vi "Mensagem.vi"(2 "error in (no error)":errorcluster, 3 "tamanho":i32) -> (0 "error IO":errorcluster, 1 "Mensagem":refnum<class "Mensagem.lvclass">)   [LabVIEW 2016, in "Mensagem.lvclass"]
uses:
  Mensagem.lvclass
  Mensagem.lvclass/Mensagem.ctl
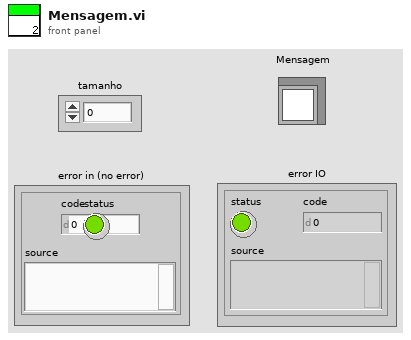
[diagram p1: front panel]
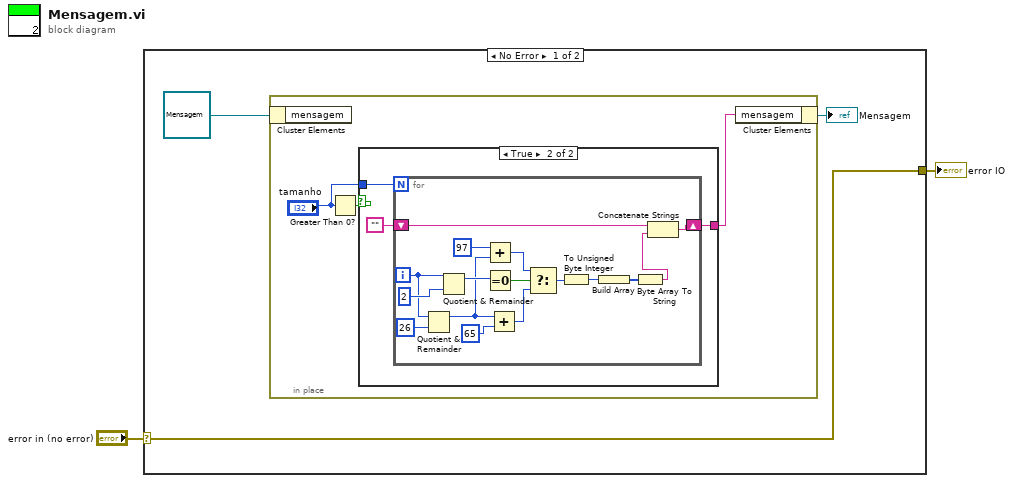
[diagram p0: block diagram]
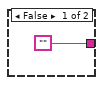
[diagram p2: hidden frame]
diagram:
  n1 = case shown="No Error" "error in (no error)" {
    selector: "error in (no error)" -> [w5 w29]
    tunnel: [w5 w29] -> w2
    frame No Error {
      n2 = in-place {
        n3 = in-place-cluster #1(refnum<class "Mensagem.lvclass"> refnum ("Mensagem.lvclass")) -> ()  [unwired: 1 out]
        n4 = Greater Than 0?(x="tamanho") -> (x > 0?=w7:bool)
        n5 = case shown="True" w7 {
          tunnel: "tamanho" -> [_ w11]
          tunnel: ["" w10] -> w6
          frame False {
          }
          frame True {
            n6 = for {
              N: w11 -> [_]
              shift-right: [w18] -> w10
              shift-left: "" -> [w16]
              i -> [w25]
              n7 = Quotient & Remainder(x=w25, y=26) -> (x-y*floor(x/y)=w20:i32)  [unwired: 1 out]
              n8 = Quotient & Remainder(x=w25, y=2) -> (x-y*floor(x/y)=w27:i32)  [unwired: 1 out]
              n9 = Add(x=97, y=w20) -> (x+y=w22:i32)
              n10 = Equal To 0?(x=w27) -> (x = 0?=w26:bool)
              n11 = Add(x=w20, y=65) -> (x+y=w23:i32)
              n12 = Select(t=w22, s=w26, f=w23) -> (s? t:f=w17:i32)
              n13 = To Unsigned Byte Integer(number=w17) -> (unsigned 8bit integer=w15:u8)
              n14 = Build Array(w15) -> (w14:u8[])
              n15 = Byte Array To String(unsigned byte array=w14) -> (string=w13:string)
              n16 = Concatenate Strings(w16, w13) -> (w18:string)
            }
          }
        }
        n17 = in-place-cluster #1("mensagem"=w6) -> (→"Mensagem":refnum<class "Mensagem.lvclass">)
      }
    }
    frame Error {
    }
  }
  "error IO" <- w2
